vi "Acquire.vi"(8 "error in (no error)":T3 caption="entrée d'erreur (pas d'erreur)", 9 "File d'attente de données":refnum<queue>, 10 "Notificateur de données":refnum<notifier>, 11 "Ressources matérielles en entrée":T1) -> (0 "error out":T3 caption="sortie d'erreur", 3 "Ressources matérielles en sortie":T1)   [LabVIEW 2020, in "Acquisition.lvlib"]
doc: "Effectuez l'acquisition. Remplacez le contenu de ce diagramme par des appels au matériel d'acquisition."
uses:
  Acquisition.lvlib
  Hardware Configuration.ctl
  Signal Type.ctl
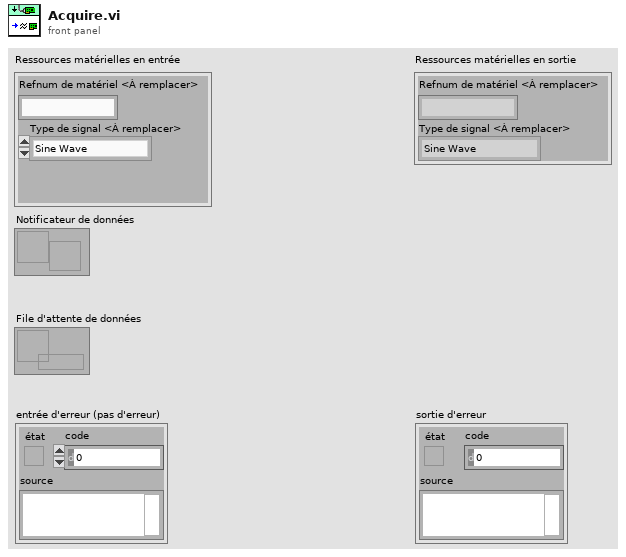
[diagram p1: front panel]
types:
  T1 = typedef "Acquisition.lvlib/Hardware Configuration.ctl" = cluster{"Refnum de matériel <À remplacer>":string, "Type de signal <À remplacer>":T2}
  T2 = typedef "Acquisition.lvlib/Signal Type.ctl" = enum16{"Sine Wave", "Square with Noise", "Signal triangulaire", "Simulation DAQ"}
  T3 = cluster{"état":bool, "code":i32, "source":string}
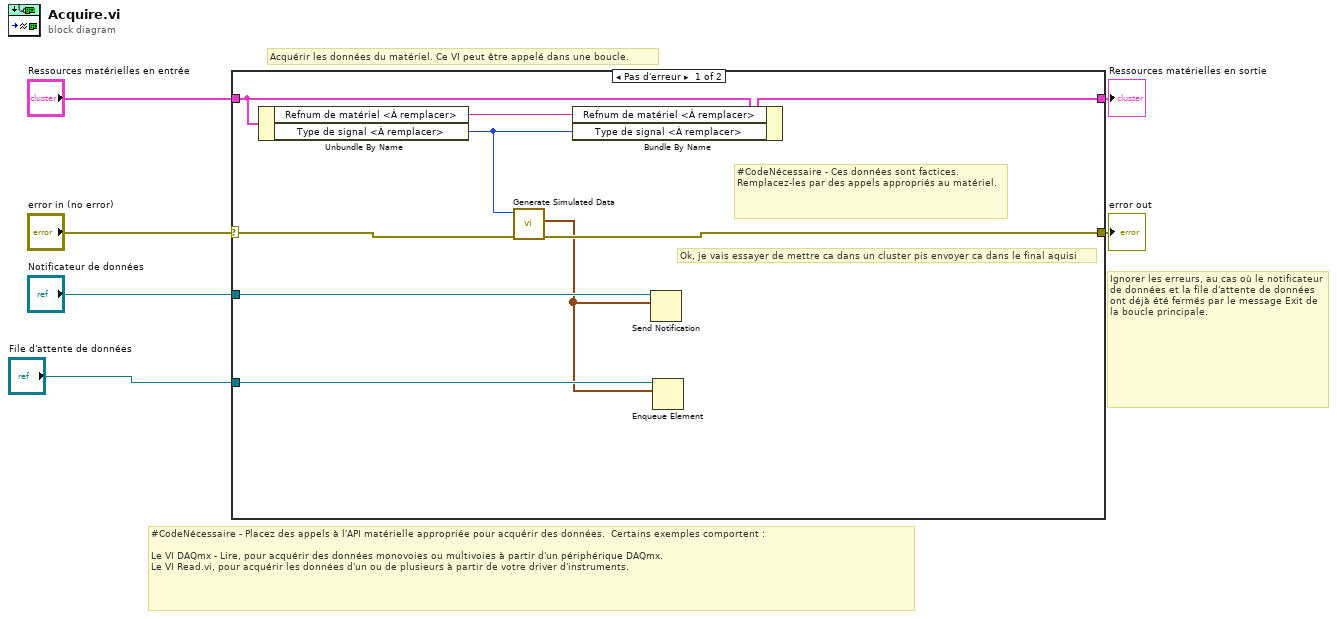
[diagram p0: block diagram]
diagram:
  # "Ignorer les erreurs, au cas où le notificateur de données et la file d'attente de données ont déjà été fermés par le message Exit de la boucle principale."
  # "Acquérir les données du matériel. Ce VI peut être appelé dans une boucle."
  # "#CodeNécessaire - Placez des appels à l'API matérielle appropriée pour acquérir des données.  Certains exemples comportent :\n\nLe VI DAQmx - Lire, pour acquérir des données monovoies ou multivoies à partir d'un périphérique DAQmx.\nLe VI Read.vi, pour acquérir les données d'un ou de plusieurs à partir de votre driver d'instruments."
  n1 = case shown="Pas d'erreur" "error in (no error)" {
    selector: "error in (no error)" -> [w14 w16]
    tunnel: "Ressources matérielles en entrée" -> [w11 w17]
    tunnel: [w15 w17] -> w4
    tunnel: "File d'attente de données" -> [w10 _]
    tunnel: [w9 w16] -> w2
    tunnel: "Notificateur de données" -> [w8 _]
    frame No Error {
      # "Ok, je vais essayer de mettre ca dans un cluster pis envoyer ca dans le final aquisi"
      # "#CodeNécessaire - Ces données sont factices. Remplacez-les par des appels appropriés au matériel."
      n2 = Unbundle By Name(w11) -> ("Refnum de matériel <À remplacer>"=w12:string, "Type de signal <À remplacer>"=w13:T2)
      n3 = call "Generate Simulated Data.vi"("error in (no error)"=w14, "Type de signal"=w13) -> ("error out"=w9:T3, "Données du graphe"=w7:waveform(dbl)[])  [unwired: 8 in]
      n4 = Bundle By Name(cluster=w11, "Refnum de matériel <À remplacer>"=w12, "Type de signal <À remplacer>"=w13) -> (w15:T1)
      n5 = Send Notification(notification=w7, notifier=w8) -> ()  [unwired: 1 in, 2 out]
      n6 = Enqueue Element(queue=w10, element=w7) -> ()  [unwired: 2 in, 3 out]
    }
    frame Error {
    }
  }
  "Ressources matérielles en sortie" <- w4
  "error out" <- w2
